vi "drop table.vi"(8 "error in (no error)":errorcluster, 10 "table":string, 11 "database":string="database1.mdb") -> (0 "error out":errorcluster)   [LabVIEW 2016, in "数据查询.lvlib"]
uses:
  <vilib>/addons/database/Connection.llb/DB Tools Open Connec (String).vi
  <vilib>/addons/database/NI_Database_API.lvlib
  database/Access/Access Lib.lvlib
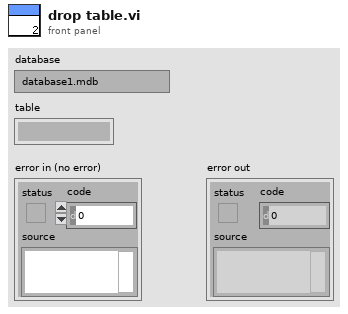
[diagram p1: front panel]
types:
  T1 = typedef "NI_Database_API.lvlib/Conn ObjectReference.ctl" = refnum<k1>
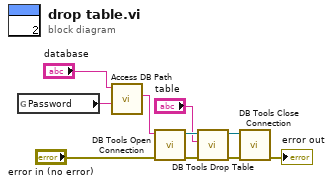
[diagram p0: block diagram]
diagram:
  n1 = global read "外部调用接口全局变量.vi" "Password"() -> (w2:string)
  n2 = call "Access DB Path.vi"("Password"=w2, "database"="database") -> ("Connection information"=w3:string)  [unwired: 8 in, 1 out]
  n3 = call-poly <vilib>:"DB Tools Open Connection.vi"("error in (no error)"="error in (no error)", "connection information"=w3) -> ("error out"=w8:errorcluster, "connection reference"=w10:T1)  [unwired: 6 in]
  n4 = call <vilib>:"DB Tools Drop Table.vi"("error in (no error)"=w8, "table"="table", "connection reference"=w10) -> ("error out"=w7:errorcluster, "connection reference out"=w9:T1)  [unwired: 5 in]
  n5 = call <vilib>:"DB Tools Close Connection.vi"("error in (no error)"=w7, "connection reference"=w9) -> ("error out"=→"error out":errorcluster)  [unwired: 5 in]
